vi "Start Live Mode.vi"(8 "error in (no error)":errorcluster, 10 "Camera Settings":T1={"Exposure Time (ms)"=100.0, "Binning"=enum."2x2", "Scan Mode"=0, "Frames to Acquire"=1000.0, "Pixel Correction"=FALSE, "Frames to Skip"=0, "File Path"=path "", "Duty cycle"=0.0, "ALEX"=FALSE, "Shutter Enable"=[], "Timelapse Interval (s)"=0, "fluidics trigger frame"=0} {"Timelapse Interval (s)" max=60000 step=1; "Exposure Time (ms)" min=1.0 max=10000.0 step=1.0}, 11 "Orca-Flash 4.0 V2 in":refnum<class "Hamamatsu Camera.lvclass">) -> (0 "error out":errorcluster, 3 "Orca-Flash 4.0 V2 out":refnum<class "Hamamatsu Camera.lvclass">)   [LabVIEW 2018, in "Hamamatsu Camera.lvlib" / "Hamamatsu Camera.lvclass"]
uses:
  Hamamatsu Camera.lvclass
  C:/FlashGordon/Development/Hardware/Camera/Camera.lvclass
  Resources/Type Defs/Camera Settings.ctl
  Resources/GLOBAL/GLOBAL Time-critical.vi
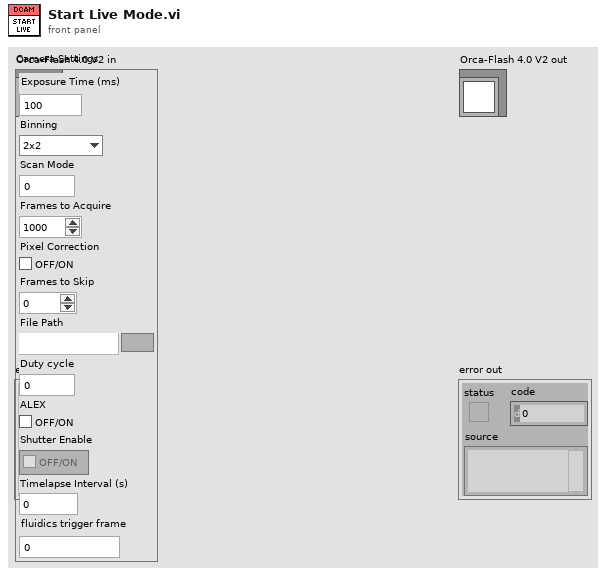
[diagram p1: front panel]
types:
  T1 = typedef "Camera Settings.ctl" = cluster{"Exposure Time (ms)":dbl, "Binning":enum16{"1x1", "2x2", "4x4"}, "Scan Mode":i32, "Frames to Acquire":dbl, "Pixel Correction":bool, "Frames to Skip":u32, "File Path":path, "Duty cycle":dbl, "ALEX":bool, "Shutter Enable":bool[], "Timelapse Interval (s)":u32, "fluidics trigger frame":u16}
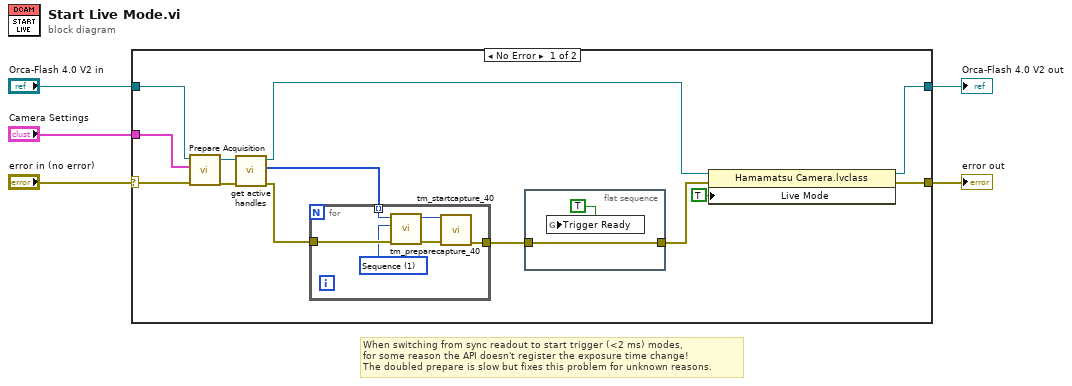
[diagram p0: block diagram]
diagram:
  # "When switching from sync readout to start trigger (<2 ms) modes,\nfor some reason the API doesn't register the exposure time change!\nThe doubled prepare is slow but fixes this problem for unknown reasons."
  n1 = case shown="No Error" "error in (no error)" {
    selector: "error in (no error)" -> [w11 w28]
    tunnel: [w17 w27] -> w5
    tunnel: [w16 w28] -> w4
    tunnel: "Orca-Flash 4.0 V2 in" -> [w15 w27]
    tunnel: "Camera Settings" -> [w12 _]
    frame No Error {
      n2 = call "Prepare Acquisition.vi"("error in (no error)"=w11, "Flash Settings"=w12, "Orca-Flash 4.0 in"=w15) -> ("error out"=w6:errorcluster, "Orca-Flash 4.0 out"=w7:refnum<class "Hamamatsu Camera.lvclass">)  [unwired: 7 in]
      n3 = call-dynamic "get active handles.vi"("error in (no error)"=w6, "Hamamatsu Camera in"=w7) -> ("error out"=w8:errorcluster, "Handles"=w10:u32[], "Hamamatsu Camera out"=w9:refnum<class "Hamamatsu Camera.lvclass">)  [unwired: 5 in, 2 out]
      n4 = for {
        tunnel: w8 -> [w24]
        tunnel: w10 -> [w23] mode=indexing
        tunnel: [w21] -> w14
        w22 = 1 items=["Snap", "Sequence"] ("Capture mode")
        n5 = call <userlib>:"tm_preparecapture_40.vi"("error in (no error)"=w24, "Capture mode"=w22, "Handle in"=w23) -> ("error out"=w26:errorcluster, "Handle out"=w25:u32)  [unwired: 5 in, 2 out]
        n6 = call <userlib>:"tm_startcapture_40.vi"("error in (no error)"=w26, "Handle in"=w25) -> ("error out"=w21:errorcluster)  [unwired: 8 in, 1 out]
      }
      n7 = flat-sequence {
        tunnel: w14 -> [w20]
        tunnel: [w20] -> w13
        frame #0 {
          n8 = global write "GLOBAL Time-critical.vi" "Trigger Ready"(TRUE ("new element/subarray")) -> ()
        }
      }
      n9 = property class="Hamamatsu Camera.lvclass"(reference=w9, error in=w13, "Live Mode"=TRUE) -> (reference out=w17:refnum<class "Hamamatsu Camera.lvclass">, error out=w16:errorcluster)
    }
    frame Error {
    }
  }
  "error out" <- w4
  "Orca-Flash 4.0 V2 out" <- w5
